vi "Window.vi"(1 "Normalize? (False)":bool, 2 "N":i32, 3 "window type":T1) -> (0 "window":dbl[](array[numeric]))   [LabVIEW 2020]
uses:
  Window Type.ctl
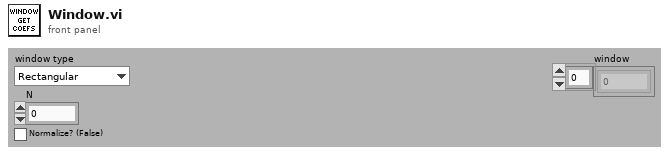
[diagram p1: front panel]
types:
  T1 = typedef "Window Type.ctl" = enum16{"Rectangular", "Hanning", "Blackman-Harris"}
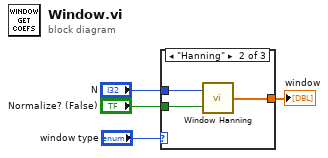
[diagram p0: block diagram]
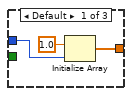
[diagram p2: hidden frame]
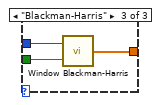
[diagram p3: hidden frame]
diagram:
  n1 = case shown="\"Hanning\"" "window type" {
    tunnel: "N" -> [w7 w10 w13]
    tunnel: "Normalize? (False)" -> [_ w9 w12]
    tunnel: [w6 w8 w11] -> w1
    frame Default {
      n2 = Initialize Array(1.0, w7) -> (w6:dbl[])
    }
    frame "Hanning" {
      n3 = call "Window Hanning.vi"("Normalize? (False)"=w9, "N"=w10) -> ("window"=w8:dbl[])
    }
    frame "Blackman-Harris" {
      n4 = call "Window Blackman-Harris.vi"("Normalize? (False)"=w12, "N"=w13) -> ("window"=w11:dbl[])
    }
  }
  "window" <- w1
